vi "Zero Delete Complex.vi"(1 "P":cdb[](array[numeric]) format="%.2f") -> (0 "Q":cdb[](array[numeric]) format="%.2f")   [LabVIEW 2017, in "NI_AdvCtrl_continuous linear.lvlib"]
doc: "LabVIEW no longer supports this VI. You can obtain similar functionality by installing the LabVIEW Simulation Module."
uses:
  <vilib>/addons/control/advanced/NI_AdvCtrl_continuous linear.lvlib
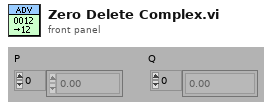
[diagram p1: front panel]
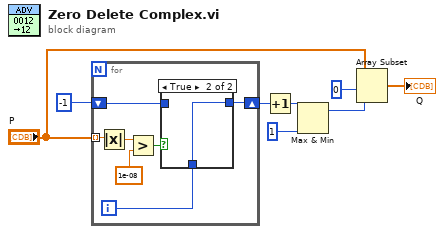
[diagram p0: block diagram]
diagram:
  n1 = for {
    tunnel: "P" -> [w15] mode=indexing
    shift-right: [w10] -> w6
    shift-left: -1 -> [w9]
    i -> [w11]
    n2 = Absolute Value(x=w15) -> (abs(x)=w14:dbl)
    n3 = Greater?(x=w14, y=1e-08) -> (0:w12:bool)
    n4 = case shown="True" w12 {
      tunnel: w11 -> [_ w17]
      tunnel: [w16 w17] -> w10
      tunnel: w9 -> [w16 _]
      frame False {
      }
      frame True {
      }
    }
  }
  n5 = Increment(x=w6) -> (x+1=w3:i32)
  n6 = Max & Min(x=w3, y=1) -> (max(x,y)=w2:i32)  [unwired: 1 out]
  n7 = Array Subset(array="P", index=0, length=w2) -> (→"Q":cdb[])
